vi "ProdaNG.GetWabcoNumbers.vi"(7 "systemName":string, 8 "error in (no error)":errorcluster, 10 "Production Line":string, 11 "dbHandle":i32) -> (0 "error out":errorcluster, 1 "WabcoPartIDs":T1[](array[typedef]), 2 "WabcoParts":T2[](array[typedef]), 3 "dbHandle":i32)   [LabVIEW 2016]
doc: "This function returns a product structure for a product, which is identified by a part and a serial number.\nImportant information: The field 'individual' was taken over from the field 'allgemein' of the legacy data directly. Because of this most products have the value 0 further on and only a few the value 1. \nParameter:\nhandle is an Integer, which is returned by the function Login() at the creation of a new connection.\nwabcoPartId is the Id of the part.\nserialNumber is the serial number of the product for the part above.\nproduct is a pointer on a product structure, which is filled if the returncode is 0. The structure must be defined in the calling program.\n\nReturncodes:\n0 No error\n< 0 ORACLE Error code\n6 (ERROR_INVALID_HANDLE) in case of an invalid handle\n1403 Record does not exist"
uses:
  Controls/ProdaNG.WabcoPart.ctl
  Controls/ProdaNG.Identification.ctl
  Configurator/ProdaNG.Configurator.Glb.vi
panel:
  out "Total":i32
  out "Idx":i32
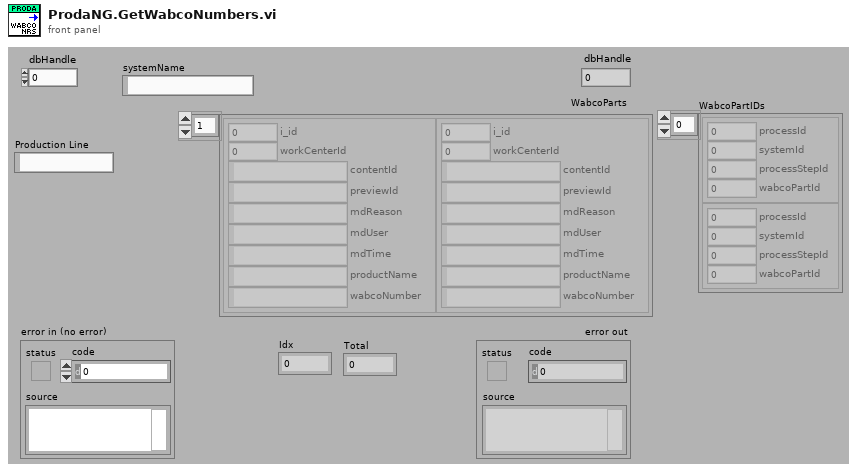
[diagram p1: front panel]
types:
  T1 = typedef "ProdaNG.Identification.ctl" = cluster{"processId":i32, "systemId":i32, "processStepId":i32, "wabcoPartId":i32}
  T2 = typedef "ProdaNG.WabcoPart.ctl" = cluster{"i_id":i32, "workCenterId":i32, "contentId":string, "previewId":string, "mdReason":string, "mdUser":string, "mdTime":string, "productName":string, "wabcoNumber":string}
  T3 = typedef "ProdaNG.ProdutionLine.ctl" = cluster{"i_id":i32, "description":string}
  T4 = typedef "ProdaNG.Process.ctl" = cluster{"i_id":i32, "productionLineId":i32, "releaseId":i32, "contentId":string, "previewId":string, "mdReason":string, "mdUser":string, "mdTime":string, "description":string}
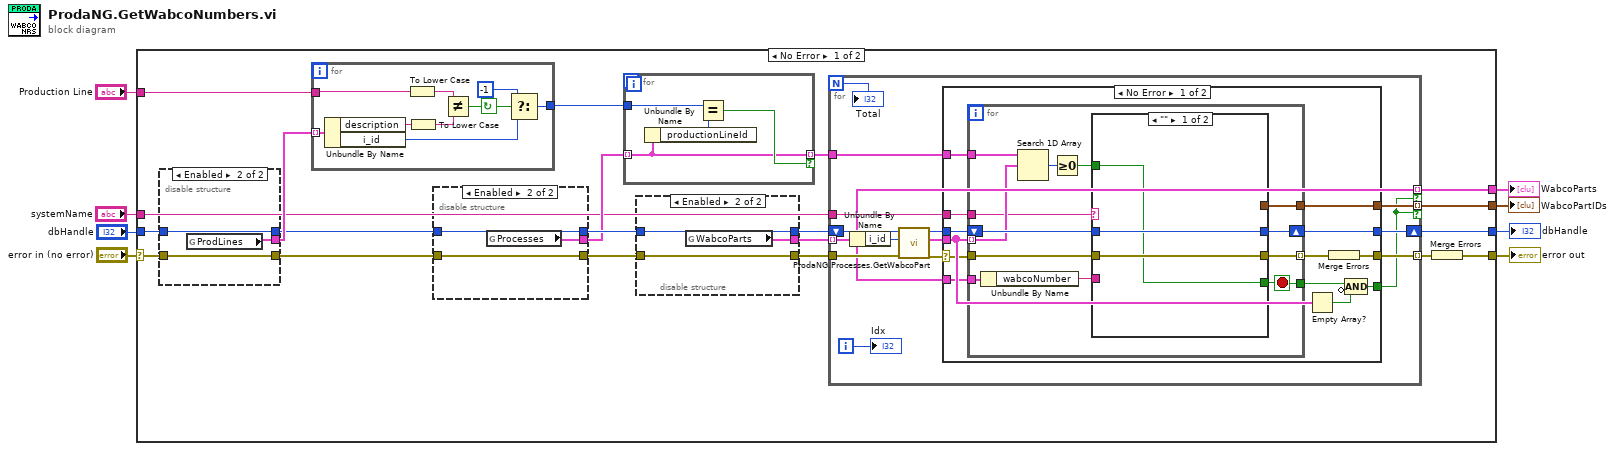
[diagram p0: block diagram]
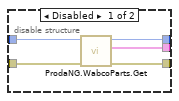
[diagram p2: hidden frame]
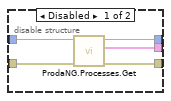
[diagram p3: hidden frame]
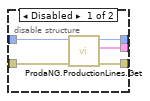
[diagram p4: hidden frame]
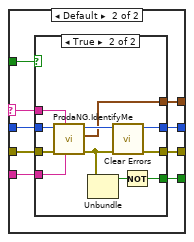
[diagram p5: hidden frame]
diagram:
  n1 = case shown="No Error" "error in (no error)" {
    selector: "error in (no error)" -> [w26 w134]
    tunnel: [w18 w134] -> w7
    tunnel: "dbHandle" -> [w25 w133]
    tunnel: [w21 w133] -> w5
    tunnel: "Production Line" -> [w15 _]
    tunnel: [w17 _] -> w3
    tunnel: "systemName" -> [w10 _]
    tunnel: [w9 _] -> w1
    frame No Error {
      n2 = disable-structure shown="Enabled" {
        disable-tunnel: w26 -> [w49 w50]
        disable-tunnel: w25 -> [w48 w51]
        disable-tunnel: [w47 w52] -> w16
        disable-tunnel: [w46 w50] -> w13
        disable-tunnel: [w45 w51] -> w12
        frame Disabled {
          n3 = call "ProdaNG.ProductionLines.Get.vi"("error in (no error)"=w49, "dbHandleIn"=w48) -> ("error out"=w46:errorcluster, "ProdLines"=w47:T3[], "dbHandle"=w45:i32)  [unwired: 7 in]
        }
        frame Enabled {
          n4 = global read "ProdaNG.Configurator.Glb.vi" "ProdLines"() -> (w52:T3[])
        }
      }
      n5 = for {
        tunnel: w16 -> [w61] mode=indexing
        tunnel: w15 -> [w59]
        tunnel: [w53] -> w14
        stop <- w56 continue-if-true
        n6 = Unbundle By Name(w61) -> ("description"=w60:string, "i_id"=w55:i32)
        n7 = To Lower Case(string=w59) -> (all lower case string=w58:string)
        n8 = To Lower Case(string=w60) -> (all lower case string=w57:string)
        n9 = Not Equal?(x=w58, y=w57) -> (x != y?=w56:bool)
        n10 = Select(t=-1, s=w56, f=w55) -> (s? t:f=w53:i32)
      }
      n11 = disable-structure shown="Enabled" {
        disable-tunnel: [w41 w43] -> w28
        disable-tunnel: [w40 w42] -> w27
        disable-tunnel: [w39 w44] -> w24
        disable-tunnel: w13 -> [w38 w42]
        disable-tunnel: w12 -> [w37 w43]
        frame Disabled {
          n12 = call "ProdaNG.Processes.Get.vi"("error in (no error)"=w38, "dbHandleIn"=w37) -> ("error out"=w40:errorcluster, "Processes"=w39:T4[], "dbHandle"=w41:i32)  [unwired: 7 in]
        }
        frame Enabled {
          n13 = global read "ProdaNG.Configurator.Glb.vi" "Processes"() -> (w44:T4[])
        }
      }
      n14 = for {
        tunnel: w24 -> [w130] mode=indexing
        tunnel: [w130] -> w20 mode=indexing if=w131
        tunnel: w14 -> [w129]
        n15 = Unbundle By Name(w130) -> ("productionLineId"=w132:i32)
        n16 = Equal?(x=w129, y=w132) -> (x = y?=w131:bool)
      }
      n17 = disable-structure shown="Enabled" {
        disable-tunnel: w28 -> [w33 w35]
        disable-tunnel: w27 -> [w32 w34]
        disable-tunnel: [w31 w34] -> w23
        disable-tunnel: [w30 w35] -> w22
        disable-tunnel: [w29 w36] -> w11
        frame Disabled {
          n18 = call "ProdaNG.WabcoParts.Get.vi"("error in (no error)"=w32, "dbHandleIn"=w33) -> ("error out"=w31:errorcluster, "WabcoParts"=w29:T2[], "dbHandle"=w30:i32)  [unwired: 7 in]
        }
        frame Enabled {
          n19 = global read "ProdaNG.Configurator.Glb.vi" "WabcoParts"() -> (w36:T2[])
        }
      }
      n20 = for {
        N -> [w62]
        tunnel: w11 -> [w65] mode=indexing
        tunnel: w23 -> [w76]
        shift-right: [w71] -> w21
        shift-left: w22 -> [w74]
        tunnel: w20 -> [w73]
        tunnel: [w65] -> w17 mode=indexing if=w66
        tunnel: [w69] -> w19 mode=indexing
        tunnel: w10 -> [w70]
        tunnel: [w68] -> w9 mode=indexing if=w66
        i -> [w63]
        n21 = Unbundle By Name(w65) -> ("i_id"=w75:i32)
        n22 = call "ProdaNG.Processes.GetWabcoPart.vi"("error in (no error)"=w76, "wabcoPartId"=w75, "dbHandleIn"=w74) -> ("error out"=w64:errorcluster, "Processes"=w67:T4[], "dbHandle"=w72:i32)  [unwired: 6 in]
        n23 = case shown="No Error" w64 {
          selector: w64 -> [w77 w128]
          tunnel: w73 -> [w89 _]
          tunnel: w72 -> [w88 w127]
          tunnel: [w87 w127] -> w71
          tunnel: w70 -> [w85 _]
          tunnel: [w84 w128] -> w69
          tunnel: [w83 _] -> w68
          tunnel: w67 -> [w80 _]
          tunnel: [w79 _] -> w66
          tunnel: w65 -> [w78 _]
          frame No Error {
            n24 = for {
              tunnel: w89 -> [w102]
              tunnel: w80 -> [w97] mode=indexing
              shift-right: [w99] -> w87
              shift-left: w88 -> [w100]
              tunnel: w77 -> [w98]
              tunnel: [w96] -> w86 mode=indexing
              tunnel: w85 -> [w90]
              tunnel: [w93] -> w83
              tunnel: [w92] -> w82
              tunnel: w78 -> [w91]
              stop <- w92 stop-if-true
              n25 = Unbundle By Name(w91) -> ("wabcoNumber"=w95:string)
              n26 = Search 1D Array(1D array=w102, element=w97) -> (index of element=w101:i32)  [unwired: 1 in]
              n27 = Greater Or Equal To 0?(x=w101) -> (x >= 0?=w94:bool)
              n28 = case shown="\"\"" w90 {
                selector: w90 -> [_ w106]
                tunnel: w100 -> [w104 w114]
                tunnel: [w104 w113] -> w99
                tunnel: w98 -> [w105 w112]
                tunnel: [w105 w111] -> w96
                tunnel: w95 -> [_ w110]
                tunnel: w94 -> [w103 w109]
                tunnel: [_ w108] -> w93
                tunnel: [w103 w107] -> w92
                frame "" {
                }
                frame Default {
                  n29 = case shown="True" w109 {
                    tunnel: w114 -> [w116 w126]
                    tunnel: [w116 w125] -> w113
                    tunnel: w112 -> [w115 w124]
                    tunnel: [w115 w118] -> w111
                    tunnel: w110 -> [_ w123]
                    tunnel: w106 -> [_ w122]
                    tunnel: [_ w119] -> w107
                    tunnel: [_ w117] -> w108
                    frame False {
                    }
                    frame True {
                      n30 = call "ProdaNG.IdentifyMe.vi"("wabcoNumber"=w123, "systemName"=w122, "error in"=w124, "dbHandleIn"=w126) -> ("error out"=w121:errorcluster, "Identification"=w117:T1, "dbHandle"=w125:i32)  [unwired: 5 in]
                      n31 = Unbundle(w121) -> ("status"=w120:bool)  [unwired: 2 out]
                      n32 = call <vilib>:"Clear Errors.vi"("error in (no error)"=w121) -> ("error out"=w118:errorcluster)  [unwired: 5 in, 1 out]
                      n33 = Not(x=w120) -> (.not. x?=w119:bool)
                    }
                  }
                }
              }
            }
            n34 = Empty Array?(array=w80) -> (empty?=w81:bool)
            n35 = Merge Errors(w86) -> (w84:errorcluster)
            n36 = Compound Arithmetic op=AND(w82, invert w81) -> (w79:bool)
          }
          frame Error {
          }
        }
        "Idx" <- w63
        "Total" <- w62
      }
      n37 = Merge Errors(w19) -> (w18:errorcluster)
    }
    frame Error {
    }
  }
  "error out" <- w7
  "dbHandle" <- w5
  "WabcoParts" <- w3
  "WabcoPartIDs" <- w1
